vi "DisplayCross.vi"(9 "CorrectAnswer":bool, 10 "Grid":T1, 11 "new picture in":picture) -> (3 "new picture out":picture)   [LabVIEW 2020]
panel:
  out "new picture":picture
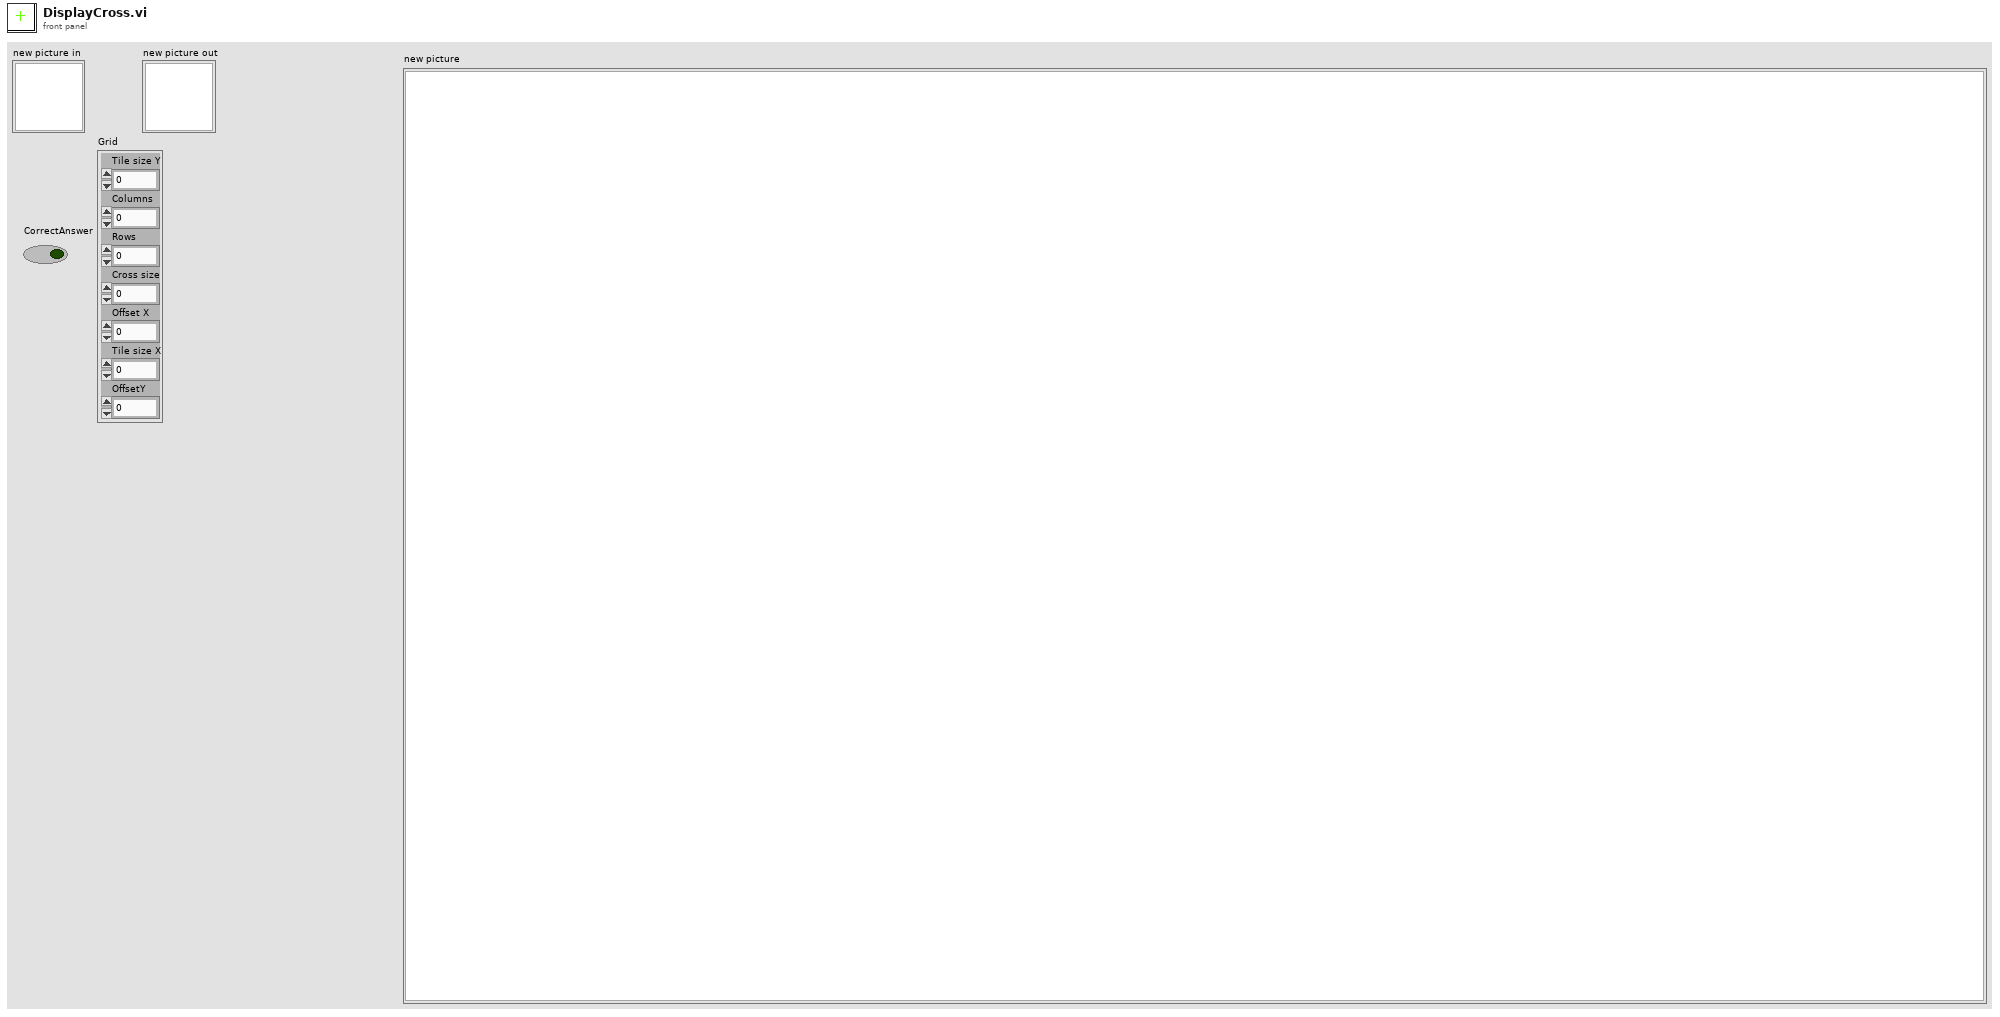
[diagram p1: front panel]
types:
  T1 = cluster{"Tile size Y":dbl, "Columns":dbl, "Rows":dbl, "Cross size":dbl, "Offset X":dbl, "Tile size X":dbl, "OffsetY":dbl}
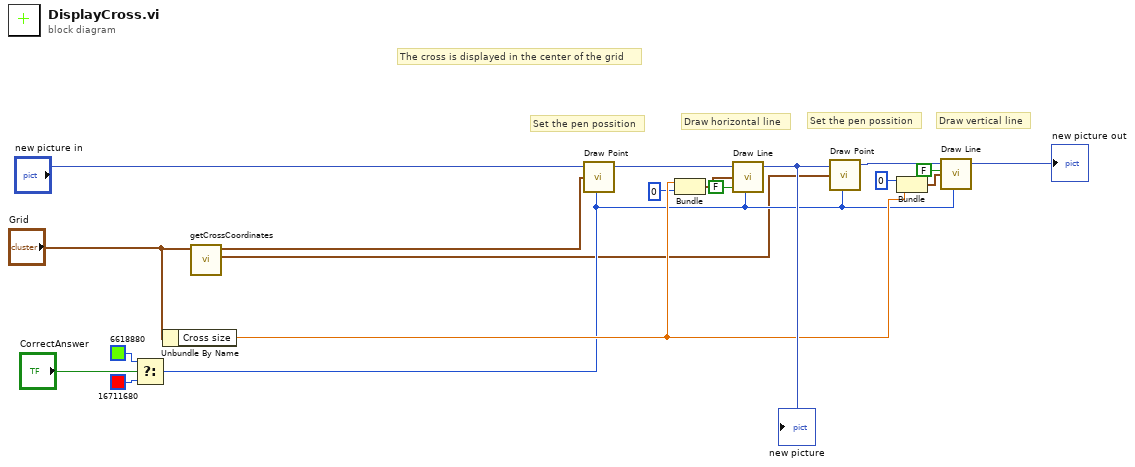
[diagram p0: block diagram]
diagram:
  # "Draw vertical line"
  # "Draw horizontal line"
  # "Set the pen possition"
  # "Set the pen possition"
  # "The cross is displayed in the center of the grid"
  n1 = Select(t=u32 6618880, s="CorrectAnswer", f=u32 16711680) -> (s? t:f=w4:u32)
  n2 = Unbundle By Name("Grid") -> ("Cross size"=w10:dbl)
  n3 = call "getCrossCoordinates.vi"("Grid"="Grid") -> ("verticalCoor"=w1:cluster{dbl, dbl}, "horizontalCoor"=w2:cluster{dbl, dbl})  [unwired: 9 in]
  n4 = call <vilib>:"Draw Point.vi"("picture"="new picture in", "point(x,y)"=w2, "color(black)"=w4) -> ("new picture"=w19:picture)  [unwired: 6 in]
  n5 = Bundle("Cross size"=w10, 0) -> (w17:cluster{"Cross size":dbl, i32})  [unwired: 1 in]
  n6 = call <vilib>:"Draw Line.vi"("picture"=w19, "end point"=w17, "absolute coordinates?(T)"=FALSE, "color(black)"=w4) -> ("new picture"=w15:picture)  [unwired: 5 in]
  "new picture" <- w15
  n7 = call <vilib>:"Draw Point.vi"("picture"=w15, "point(x,y)"=w1, "color(black)"=w4) -> ("new picture"=w14:picture)  [unwired: 6 in]
  n8 = Bundle(0, "Cross size"=w10) -> (w12:cluster{i32, "Cross size":dbl})  [unwired: 1 in]
  n9 = call <vilib>:"Draw Line.vi"("picture"=w14, "end point"=w12, "absolute coordinates?(T)"=FALSE, "color(black)"=w4) -> ("new picture"=→"new picture out":picture)  [unwired: 5 in]
